vi "get timing source.vi"(8 "error in":errorcluster, 11 "module configuration in":refnum<class "TBM module configuration.lvclass">) -> (0 "error out":errorcluster, 2 "timing source enum":T1, 3 "module configuration out":refnum<class "TBM module configuration.lvclass">)   [LabVIEW 2013, in "TBM module configuration.lvclass"]
doc: "An accessor which indicates whether or not the module is capable of generating a timing source for use with a timed loop or structure. The provided enum specifies whether a standard timing source (1 kHz, 1MHz, ...) or custom timing source must be used."
uses:
  TBM module configuration.lvclass
  timing source.ctl
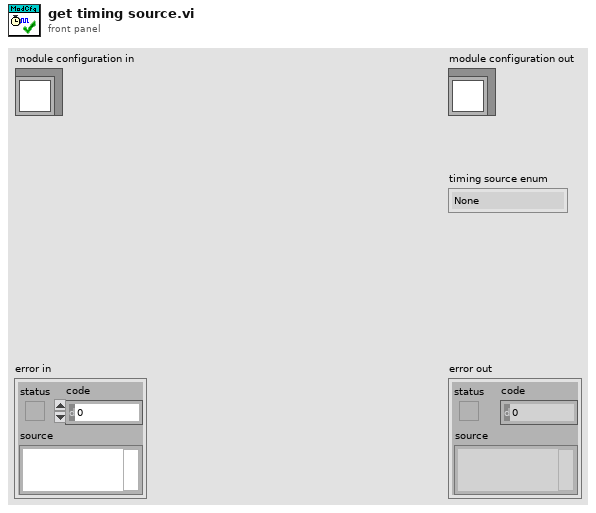
[diagram p1: front panel]
types:
  T1 = typedef "TBM module configuration.lvclass/timing source.ctl" = enum16{"None", "Custom Timing Source", "1 kHz Clock", "1 MHz Clock", "Synchronize to Scan Engine"}
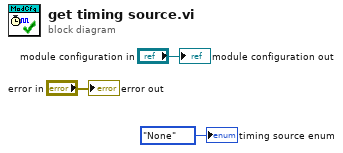
[diagram p0: block diagram]
diagram:
  "error out" <- "error in"
  "module configuration out" <- "module configuration in"
  "timing source enum" <- timing_source."None" ("timing source")
